vi "StdDev.vi"() -> ()   [LabVIEW 2017]
panel:
  out "Result":T1(plugin-control)
  out "Source":T1(plugin-control)
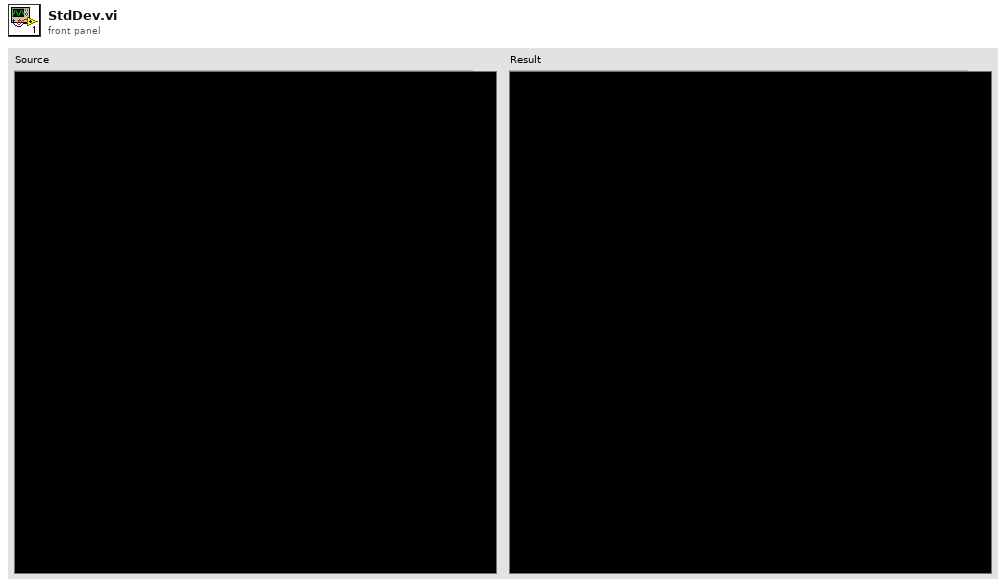
[diagram p1: front panel]
types:
  T1 = typedef "IMAQ Image.ctl" = refnum<image>
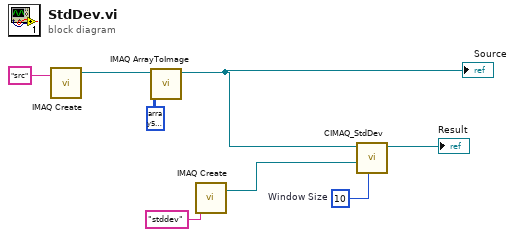
[diagram p0: block diagram]
diagram:
  w6 = 10  # Window Size
  n1 = call "IMAQ Create"("Image Name"="src") -> ("New Image"=w8:T1)  [unwired: 4 in, 1 out]
  n2 = call "IMAQ ArrayToImage"("Image Pixels (U8)"=u8[][] array514x479[246206 elements], "Image"=w8) -> ("Image Out"=w2:T1)  [unwired: 8 in, 1 out]
  "Source" <- w2
  n3 = call "IMAQ Create"("Image Name"="stddev") -> ("New Image"=w5:T1)  [unwired: 4 in, 1 out]
  n4 = call "CIMAQ_StdDev.vi"("Window Size"=w6, "Dst(optional)"=w5, "Src"=w2) -> ("Result"=→"Result":T1)  [unwired: 7 in, 1 out]
